vi "LoadSettings.vi"(8 "error in (no error)":errorcluster, 9 "new command(s)":string, 10 "DeviceName":string, 11 "Photometrics Cam v2 in":refnum<class "Photometrics_CH-250_Cam.lvclass">) -> (0 "error out":errorcluster, 2 "String":string, 3 "Photometrics Cam v2 out":refnum<class "Photometrics_CH-250_Cam.lvclass">)   [LabVIEW 2013, in "Photometrics_CH-250_Cam.lvclass"]
doc: "Load the device settings from the Database"
uses:
  Photometrics_CH-250_Cam.lvclass
  Photometrics_CH-250_Cam.lvclass/Photometrics_CH-250_Cam.ctl
  BaseDriver/BaseDriver.lvclass
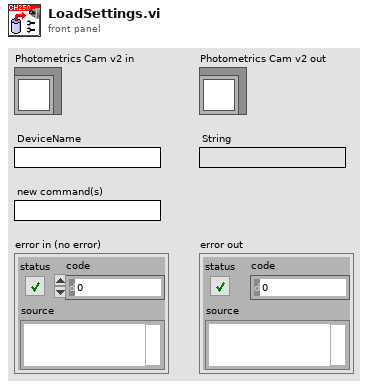
[diagram p1: front panel]
types:
  T1 = typedef "Photometrics_CH-250_Cam.lvclass/SettingsTypdef.ctl" = cluster{"trigger":T2, "gain":cluster{"Value":dbl, "Min":dbl, "Max":dbl, "StepSize":dbl, "Tolerance":dbl, "valueactual":dbl}, "Timeout":cluster{"Value":dbl, "Min":dbl, "Max":dbl, "StepSize":dbl, "Tolerance":dbl, "valueactual":dbl}, "localsavingpath":path, "save":T2, "camera name":string, "exposure":cluster{"Value":dbl, "Min":dbl, "Max":dbl, "StepSize":dbl, "Tolerance":dbl, "valueactual":dbl}, "TSetpoint":cluster{"Value":dbl, "Min":dbl, "Max":dbl, "StepSize":dbl, "Tolerance":dbl, "valueactual":dbl}, "TReading":cluster{"Value":dbl, "Min":dbl, "Max":dbl, "StepSize":dbl, "Tolerance":dbl, "valueactual":dbl}, "MaxGUIPixel":cluster{"Value":dbl, "Min":dbl, "Max":dbl, "StepSize":dbl, "Tolerance":dbl, "valueactual":dbl}, "GUIBinning":cluster{"Value":dbl, "Min":dbl, "Max":dbl, "StepSize":dbl, "Tolerance":dbl, "valueactual":dbl}, "ROI":T3, "pause":T2}
  T2 = typedef "OnOffTypeDef.ctl" = enum16{"off", "on"}
  T3 = typedef "ROI_TypDef.ctl" = cluster{"Width":cluster{"Value":dbl, "Min":dbl, "Max":dbl, "StepSize":dbl, "Tolerance":dbl, "valueactual":dbl}, "Height":cluster{"Value":dbl, "Min":dbl, "Max":dbl, "StepSize":dbl, "Tolerance":dbl, "valueactual":dbl}, "OffsetX":cluster{"Value":dbl, "Min":dbl, "Max":dbl, "StepSize":dbl, "Tolerance":dbl, "valueactual":dbl}, "OffsetY":cluster{"Value":dbl, "Min":dbl, "Max":dbl, "StepSize":dbl, "Tolerance":dbl, "valueactual":dbl}}
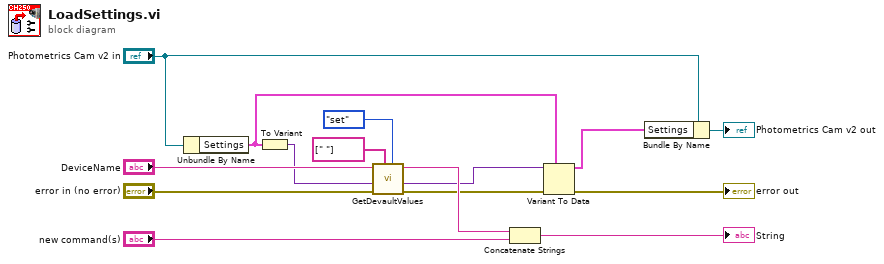
[diagram p0: block diagram]
diagram:
  n1 = Unbundle By Name("Photometrics Cam v2 in") -> ("Settings"=w4:T1)
  n2 = To Variant(anything=w4) -> (Variant=w3:variant)
  n3 = call "GetDevaultValues.vi"("set or DON'T set"=enum16{"set", "DON'T set"}."set", "set following Variables (empty = all avriables)"=string[] [" "], "error in (no error)"="error in (no error)", "variant"=w3, "Device Name"="DeviceName") -> ("error out"=w1:errorcluster, "variant out"=w5:variant, "new command(s)"=w6:string)  [unwired: 4 in]
  n4 = Concatenate Strings(w6, "new command(s)") -> (→"String":string)
  n5 = Variant To Data(error in=w1, type=w4, Variant=w5) -> (data=w15:T1, error out=→"error out":errorcluster)
  n6 = Bundle By Name(cluster="Photometrics Cam v2 in", "Settings"=w15) -> (→"Photometrics Cam v2 out":refnum<class "Photometrics_CH-250_Cam.lvclass">)
